vi "DownloadImageFromWeb.vi"(8 "error in (no error)":errorcluster, 11 "Image URL":string="http://forums.ni.com/legacyfs/online/20297_Labview-logo1.jpg") -> (0 "error out":errorcluster, 3 "Downloaded Image":T1)   [LabVIEW 2020, in "StashRoyale.lvclass"]
uses:
  StashRoyale.lvclass
  <vilib>/httpClient/LabVIEWHTTPClient.lvlib
  <vilib>/picture/picture.llb/imagedata.ctl
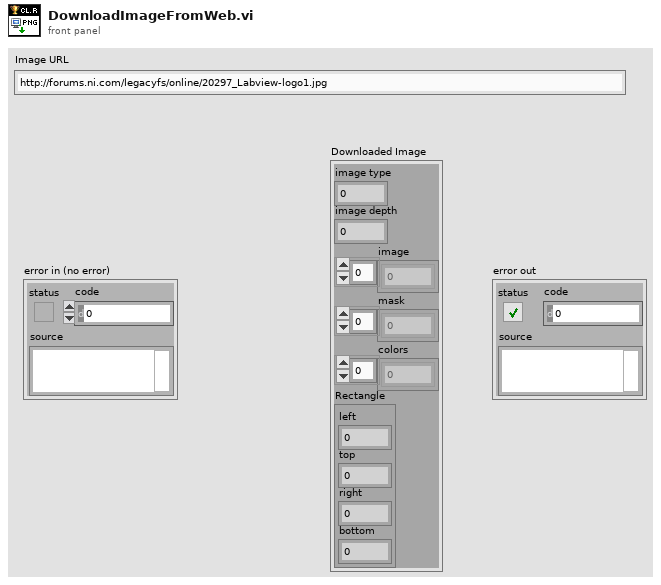
[diagram p1: front panel]
types:
  T1 = typedef "imagedata.ctl" = cluster{"image type":i32, "image depth":i32, "image":u8[], "mask":u8[], "colors":u32[], "Rectangle":cluster{"left":i16, "top":i16, "right":i16, "bottom":i16}}
  T2 = typedef "LabVIEWHTTPClient.lvlib/ClientHandle.ctl" = refnum<k1>
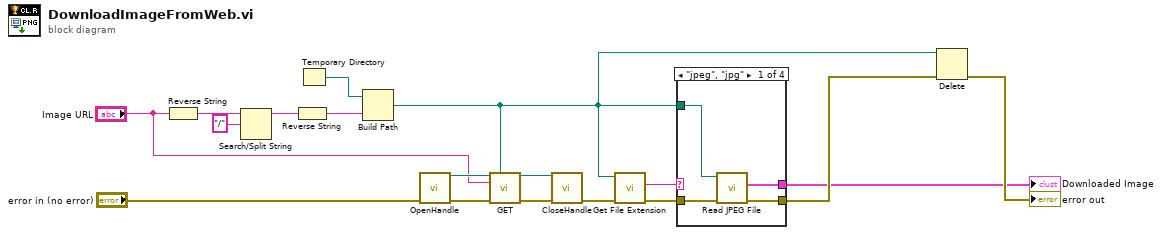
[diagram p0: block diagram]
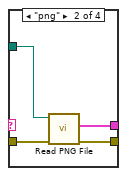
[diagram p2: hidden frame]
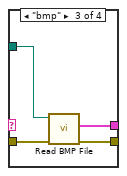
[diagram p3: hidden frame]
diagram:
  n1 = Reverse String(1:"Image URL") -> (0:w10:string)
  n2 = Search/Split String(string=w10, search string/char (-)="/") -> (substring before match=w8:string)  [unwired: 1 in, 2 out]
  n3 = Reverse String(1:w8) -> (0:w7:string)
  n4 = Temporary Directory() -> (w13:path)
  n5 = Build Path(base path=w13, name or relative path=w7) -> (appended path=w5:path)
  n6 = call <vilib>:"OpenHandle.vi"("error in (no error)"="error in (no error)") -> ("client handle out"=w18:T2, "error out"=w17:errorcluster)  [unwired: 13 in]
  n7 = call <vilib>:"GET.vi"("client handle"=w18, "output file"=w5, "url"="Image URL", "error in (no error)"=w17) -> ("client handle out"=w15:T2, "error out"=w16:errorcluster)  [unwired: 8 in, 2 out]
  n8 = call <vilib>:"CloseHandle.vi"("client handle"=w15, "error in (no error)"=w16) -> ("error out"=w12:errorcluster)  [unwired: 13 in]
  n9 = call <vilib>:"Get File Extension.vi"("error in (no error)"=w12, "file"=w5) -> ("error out"=w11:errorcluster, "lowercase file extension"=w14:string)  [unwired: 5 in, 3 out]
  n10 = case shown="\"jpeg\", \"jpg\"" w14 {
    tunnel: w5 -> [w21 w26 w27 _]
    tunnel: w11 -> [w22 w25 w30 w31]
    tunnel: [w20 w24 w29 w31] -> w6
    tunnel: [w19 w23 w28 _] -> w1
    frame "jpeg", "jpg" {
      n11 = call <vilib>:"Read JPEG File.vi"("error in (no error)"=w22, "path to JPEG file"=w21) -> ("error out"=w20:errorcluster, "image data"=w19:T1)  [unwired: 7 in, 1 out]
    }
    frame "png" {
      n12 = call <vilib>:"Read PNG File.vi"("error in (no error)"=w25, "path to PNG file"=w26) -> ("error out"=w24:errorcluster, "image data"=w23:T1)  [unwired: 7 in, 1 out]
    }
    frame "bmp" {
      n13 = call <vilib>:"Read BMP File.vi"("error in (no error)"=w30, "path to BMP file"=w27) -> ("error out"=w29:errorcluster, "image data"=w28:T1)  [unwired: 7 in, 1 out]
    }
    frame Default {
    }
  }
  "Downloaded Image" <- w1
  n14 = Delete(path (use dialog)=w5, error in=w6) -> (error out=→"error out":errorcluster)  [unwired: 3 in, 2 out]
